vi "TDMS Delete Data from Channels.vi"() -> ()   [LabVIEW 2023]
doc: "This example demonstrates how to use TDMS Delete Data Function to delete data samples of channels from TDMS File."
panel:
  out "Exists? 2":bool=TRUE
  out "Exists?":bool=TRUE
  out "wf_samples 3":i32
  out "wf_start_offset 3":dbl
  out "NI_ExpTimeStamp 3":timestamp
  out "wf_samples 4":i32
  out "wf_start_offset 4":dbl
  out "NI_ExpTimeStamp 4":timestamp
  out "Remaining data of channels \"Dev1/ai0\" and \"Dev2/ai0\"":waveform(dbl)[](graph)
  out "wf_samples":i32
  out "wf_start_offset":dbl
  out "NI_ExpTimeStamp":timestamp
  out "wf_samples 2":i32
  out "wf_start_offset 2":dbl
  out "NI_ExpTimeStamp 2":timestamp
  in  "count":i64=500
  in  "from":enum16{"start", "end"}(ring)
  in  "keep empty group/channel?":bool=TRUE
  in  "channel name(s)":T1(ring)
  out "Data written to the channels \"Dev1/ai0\" and \"Dev2/ai0\"":waveform(dbl)[](graph)
  # "Overview: Demonstrates the use of the TDMS Delete Data function to delete data samples from a .tdms file.\nInstructions:\n1. In the Data Deletion Options section, configure the data to delete from the .tdms file.\n2. Run this VI.\n3. Delete the .tdms file (located at [LabVIEW Data]\\Example Delete Data.tdms) when you are done."
  # "Data Deletion Options"
  # "Before Data Deletion"
  # "After Data Deletion"
  # "Channel \"Dev1/ai0\""
  # "Channel \"Dev1/ai0\""
  # "Channel \"Dev2/ai0\""
  # "Channel \"Dev2/ai0\""
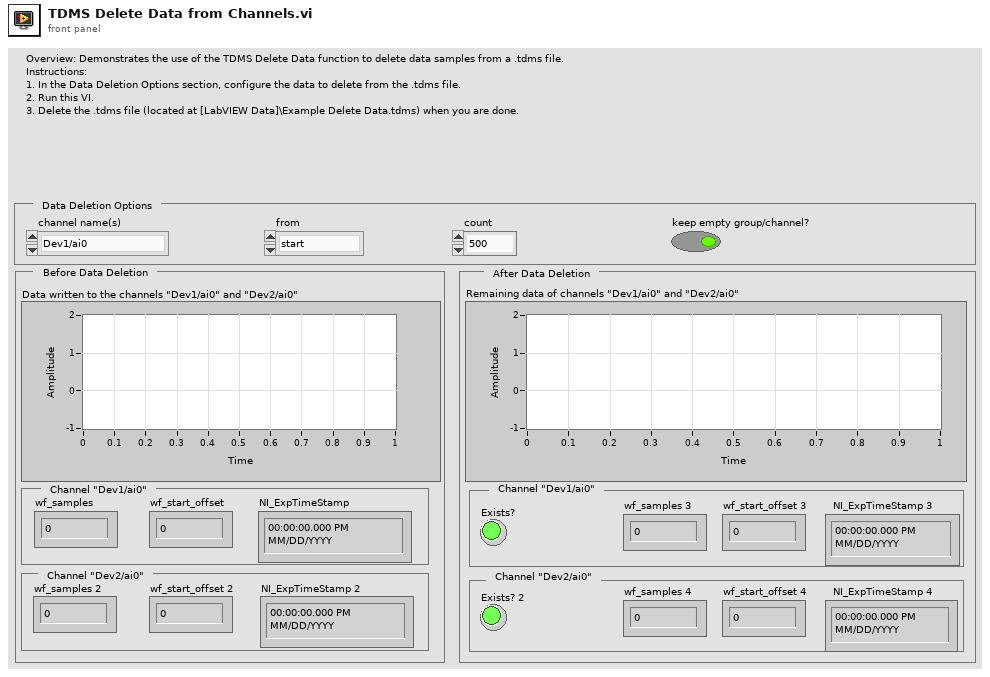
[diagram p1: front panel]
types:
  T1 = enum16{"Dev1/ai0", "Dev2/ai0", "Dev1/ai0 and Dev2/ai0"}
  T2 = enum16{"open", "open or create", "create or replace", "create", "open (read-only)"}
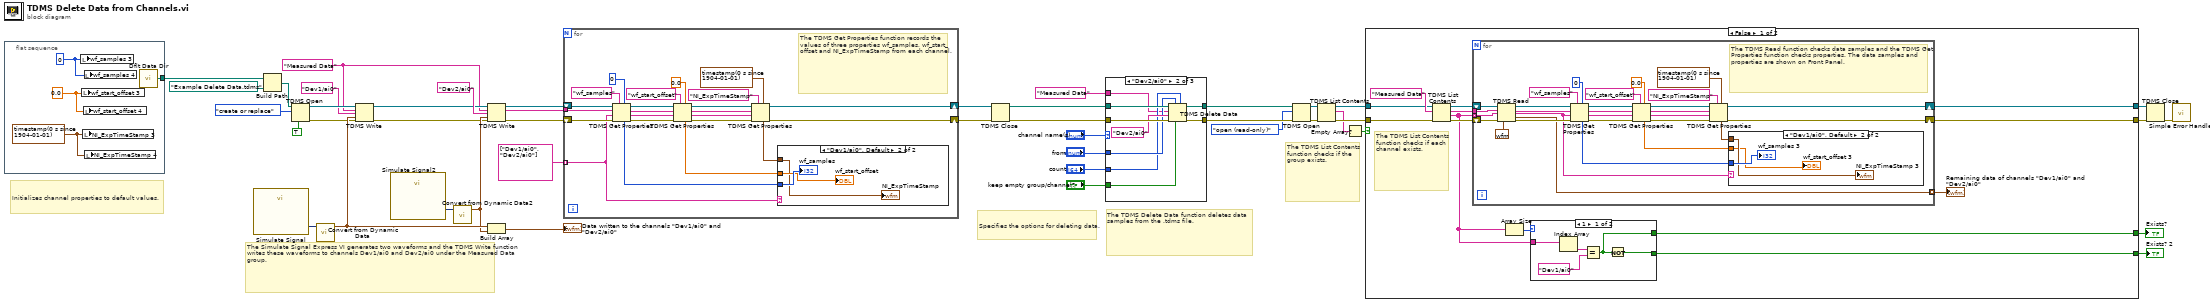
[diagram p0: block diagram]
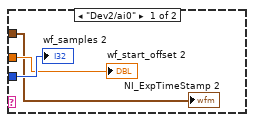
[diagram p2: hidden frame]
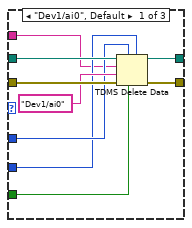
[diagram p3: hidden frame]
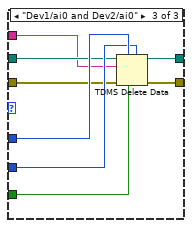
[diagram p4: hidden frame]
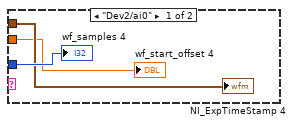
[diagram p5: hidden frame]
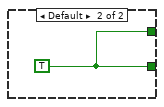
[diagram p6: hidden frame]
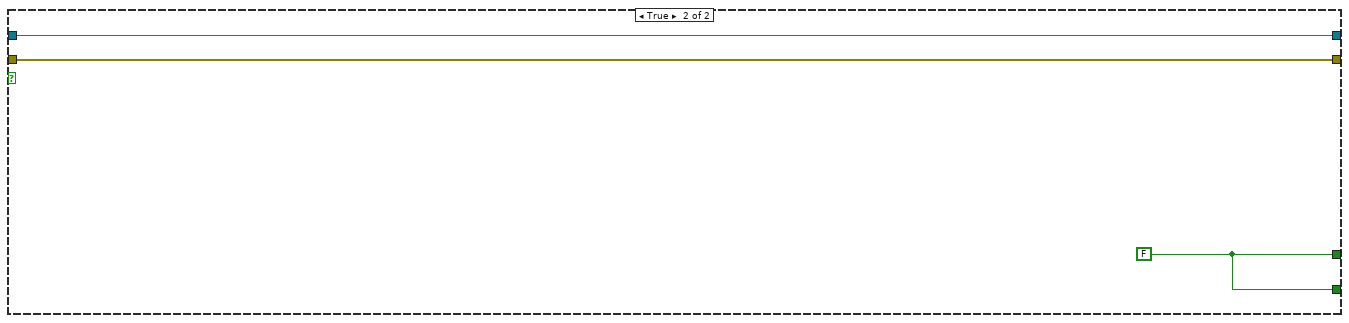
[diagram p7: hidden frame]
diagram:
  w19 = "Measured Data"
  # "The TDMS List Contents function checks if the group exists."
  # "Specifies the options for deleting data."
  # "The Simulate Signal Express VI generates two waveforms and the TDMS Write function writes these waveforms to channels Dev1/ai0 and Dev2/ai0 under the Measured Data group."
  # "The TDMS Delete Data function deletes data samples from the .tdms file."
  # "Initializes channel properties to default values."
  n1 = flat-sequence {
    tunnel: [w45] -> w6
    frame #0 {
      w46 = timestamp(0 s since 1904-01-01)
      w47 = 0.0
      w48 = 0
      n2 = local write "wf_samples 3"(w48) -> ()
      n3 = local write "wf_start_offset 3"(w47) -> ()
      n4 = local write "NI_ExpTimeStamp 3"(w46) -> ()
      n5 = local write "wf_start_offset 4"(w47) -> ()
      n6 = local write "wf_samples 4"(w48) -> ()
      n7 = local write "NI_ExpTimeStamp 4"(w46) -> ()
      n8 = call <vilib>:"Dflt Data Dir.vi"() -> ("App:Default Data Directory"=w45:path)
    }
  }
  n9 = call "Simulate Signal"() -> ("Sine"=w38:dynamicdata)  [unwired: 14 in, 1 out]
  n10 = Build Path(base path=w6, name or relative path=path "Example Delete Data.tdms" ("file path")) -> (appended path=w42:path)
  n11 = TDMS Open(6:TRUE ("disable buffering (T)"), 10:T2."create or replace" ("operation"), 11:w42) -> (0:w1:errorcluster, 3:w40:refnum<k34>)  [unwired: 4 in]
  n12 = call "Convert from Dynamic Data"("Dynamic Data Type"=w38) -> ("Waveform"=w16:waveform(dbl))  [unwired: 3 in]
  n13 = TDMS Write(0:w40, 5:w19, 7:"Dev1/ai0", 9:w16, 11:w1) -> (4:w20:refnum<k34>, 15:w2:errorcluster)  [unwired: 1 in, 2 out]
  n14 = call "Simulate Signal2"() -> ("Sine"=w31:dynamicdata)  [unwired: 14 in, 1 out]
  n15 = call "Convert from Dynamic Data2"("Dynamic Data Type"=w31) -> ("Waveform"=w5:waveform(dbl))  [unwired: 3 in]
  n16 = TDMS Write(0:w20, 5:w19, 7:"Dev2/ai0", 9:w5, 11:w2) -> (4:w29:refnum<k34>, 6:w28:string, 15:w27:errorcluster)  [unwired: 1 in, 1 out]
  n17 = Build Array(w16, w5) -> (→"Data written to the channels \"Dev1/ai0\" and \"Dev2/ai0\"":waveform(dbl)[])
  n18 = for {
    tunnel: w28 -> [w67]
    shift-right: [w65] -> w26
    shift-left: w29 -> [w68]
    shift-right: [w64] -> w25
    shift-left: w27 -> [w66]
    tunnel: string[] ["Dev1/ai0", "Dev2/ai0"] -> [w49] mode=indexing
    # "The TDMS Get Properties function records the values of three properties wf_samples, wf_start_offset and NI_ExpTimeStamp from each channel."
    n19 = TDMS Get Properties(5:0, 7:"wf_samples" ("property name"), 8:w66, 9:w49, 10:w67, 11:w68) -> (0:w59:errorcluster, 1:w60:string, 2:w61:string, 3:w62:refnum<k34>, 4:w71:i32)  [unwired: 1 out]
    n20 = TDMS Get Properties(5:0.0, 7:"wf_start_offset" ("group name in (Untitled)"), 8:w59, 9:w60, 10:w61, 11:w62) -> (0:w51:errorcluster, 1:w52:string, 2:w53:string, 3:w56:refnum<k34>, 4:w70:dbl)  [unwired: 1 out]
    n21 = TDMS Get Properties(5:timestamp(0 s since 1904-01-01), 7:"NI_ExpTimeStamp" ("group name in (Untitled)"), 8:w51, 9:w52, 10:w53, 11:w56) -> (0:w64:errorcluster, 3:w65:refnum<k34>, 4:w69:timestamp)  [unwired: 3 out]
    n22 = case shown="\"Dev1/ai0\", Default" w49 {
      tunnel: w71 -> [w74 w77]
      tunnel: w70 -> [w73 w76]
      tunnel: w69 -> [w72 w75]
      frame "Dev2/ai0" {
        "wf_samples 2" <- w74
        "wf_start_offset 2" <- w73
        "NI_ExpTimeStamp 2" <- w72
      }
      frame "Dev1/ai0", Default {
        "wf_samples" <- w77
        "wf_start_offset" <- w76
        "NI_ExpTimeStamp" <- w75
      }
    }
  }
  n23 = TDMS Close(8:w25, 11:w26) -> (0:w36:errorcluster, 3:w37:path)
  n24 = case shown="\"Dev2/ai0\"" "channel name(s)" {
    tunnel: w37 -> [w85 w95 w98]
    tunnel: w36 -> [w86 w94 w100]
    tunnel: "keep empty group/channel?" -> [w83 w90 w103]
    tunnel: "from" -> [w82 w92 w102]
    tunnel: "count" -> [w81 w91 w101]
    tunnel: [w80 w89 w99] -> w24
    tunnel: [w79 w88 w97] -> w23
    tunnel: "Measured Data" -> [w78 w87 w96]
    frame "Dev1/ai0", Default {
      n25 = TDMS Delete Data(5:w81, 6:w83, 7:w82, 8:w86, 9:"Dev1/ai0", 10:w78, 11:w85) -> (0:w80:errorcluster, 3:w79:path)
    }
    frame "Dev2/ai0" {
      n26 = TDMS Delete Data(5:w91, 6:w90, 7:w92, 8:w94, 9:"Dev2/ai0", 10:w87, 11:w95) -> (0:w89:errorcluster, 3:w88:path)
    }
    frame "Dev1/ai0 and Dev2/ai0" {
      n27 = TDMS Delete Data(5:w101, 6:w103, 7:w102, 8:w100, 10:w96, 11:w98) -> (0:w99:errorcluster, 3:w97:path)  [unwired: 1 in]
    }
  }
  n28 = TDMS Open(8:w24, 10:T2."open (read-only)" ("operation (0:open)"), 11:w23) -> (0:w12:errorcluster, 3:w13:refnum<k34>)  [unwired: 4 in]
  n29 = TDMS List Contents(4:w12, 7:w13) -> (0:w10:errorcluster, 2:w4:string[], 3:w11:refnum<k34>)  [unwired: 1 in, 1 out]
  n30 = Empty Array?(array=w4) -> (empty?=w3:bool)
  n31 = case shown="False" w3 {
    tunnel: [w105 w160] -> w15
    tunnel: w11 -> [w112 w160]
    tunnel: w10 -> [w115 w159]
    tunnel: [w116 w159] -> w9
    tunnel: [w106 w158] -> w8
    tunnel: [w107 w158] -> w7
    frame False {
      # "The TDMS List Contents function checks if each channel exists."
      n32 = TDMS List Contents(4:w115, 6:"Measured Data" ("group name"), 7:w112) -> (0:w110:errorcluster, 1:w108:string[], 2:w109:string, 3:w111:refnum<k34>)
      n33 = for {
        shift-right: [w130] -> w105
        shift-left: w111 -> [w117]
        shift-right: [w145] -> w116
        shift-left: w110 -> [w128]
        tunnel: [w124] -> w113 mode=indexing
        tunnel: w109 -> [w123]
        tunnel: w108 -> [w122] mode=indexing
        # "The TDMS Read function checks data samples and the TDMS Get Properties function checks properties. The data samples and properties are shown on Front Panel."
        n34 = TDMS Read(0:w117, 5:w123, 7:w122, 11:w128, 12:waveform(dbl) {"t0"=timestamp(0 s since 1904-01-01), "dt"=1.0, "Y"=[]} ("data type")) -> (4:w129:refnum<k34>, 6:w126:string, 8:w121:string, 10:w124:waveform(dbl), 15:w127:errorcluster)  [unwired: 3 in, 1 out]
        n35 = TDMS Get Properties(5:0, 7:"wf_samples" ("property name"), 8:w127, 9:w121, 10:w126, 11:w129) -> (0:w140:errorcluster, 1:w141:string, 2:w142:string, 3:w143:refnum<k34>, 4:w120:i32)  [unwired: 1 out]
        n36 = TDMS Get Properties(5:0.0, 7:"wf_start_offset" ("group name in (Untitled)"), 8:w140, 9:w141, 10:w142, 11:w143) -> (0:w132:errorcluster, 1:w133:string, 2:w134:string, 3:w137:refnum<k34>, 4:w118:dbl)  [unwired: 1 out]
        n37 = TDMS Get Properties(5:timestamp(0 s since 1904-01-01), 7:"NI_ExpTimeStamp" ("group name in (Untitled)"), 8:w132, 9:w133, 10:w134, 11:w137) -> (0:w145:errorcluster, 3:w130:refnum<k34>, 4:w119:timestamp)  [unwired: 3 out]
        n38 = case shown="\"Dev1/ai0\", Default" w121 {
          tunnel: w120 -> [w148 w151]
          tunnel: w119 -> [w147 w150]
          tunnel: w118 -> [w146 w149]
          frame "Dev2/ai0" {
            "wf_samples 4" <- w148
            "wf_start_offset 4" <- w146
            "NI_ExpTimeStamp 4" <- w147
          }
          frame "Dev1/ai0", Default {
            "wf_samples 3" <- w151
            "wf_start_offset 3" <- w149
            "NI_ExpTimeStamp 3" <- w150
          }
        }
      }
      "Remaining data of channels \"Dev1/ai0\" and \"Dev2/ai0\"" <- w113
      n39 = Array Size(array=w108) -> (size(s)=w104:i32)
      n40 = case shown="1" w104 {
        tunnel: [w152 w157] -> w106
        tunnel: [w156 w157] -> w107
        tunnel: w108 -> [w155 _]
        frame 1 {
          n41 = Index Array(array=w155) -> (element=w154:string)  [unwired: 1 in]
          n42 = Equal?(x=w154, y="Dev1/ai0") -> (x = y?=w152:bool)
          n43 = Not(x=w152) -> (.not. x?=w156:bool)
        }
        frame Default {
          w157 = TRUE
        }
      }
    }
    frame True {
      w158 = FALSE
    }
  }
  "Exists?" <- w8
  "Exists? 2" <- w7
  n44 = TDMS Close(8:w9, 11:w15) -> (0:w14:errorcluster)  [unwired: 1 out]
  n45 = call <vilib>:"Simple Error Handler.vi"("error in (no error)"=w14) -> ()  [unwired: 2 in, 7 out]
